vi "dllpathselect.vi"() -> (3 "appended path":path)   [LabVIEW 2025]
panel:
  out "number of replacements":i32
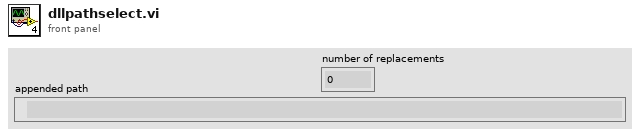
[diagram p1: front panel]
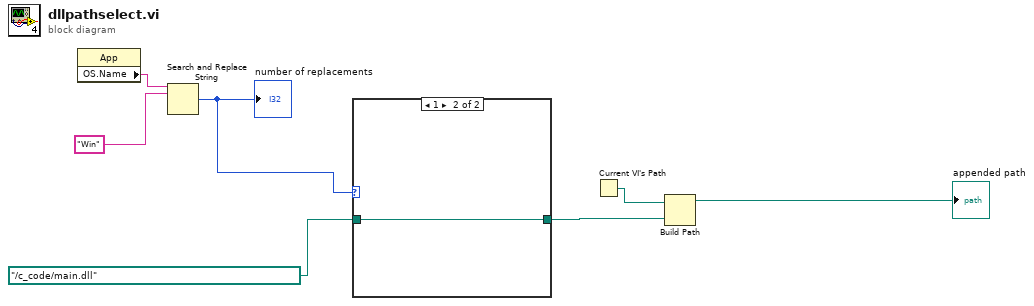
[diagram p0: block diagram]
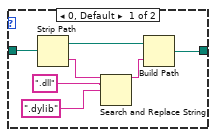
[diagram p2: hidden frame]
diagram:
  n1 = property class="App"() -> ("OS.Name"=w5:string)  [unwired: 2 in, 2 out]
  n2 = Search and Replace String(input string=w5, search string="Win") -> (number of replacements=w2:i32)  [unwired: 6 in, 3 out]
  "number of replacements" <- w2
  n3 = case shown="1" w2 {
    tunnel: path "../c_code/main.dll" ("name or relative path") -> [w14 w15]
    tunnel: [w8 w15] -> w3
    frame 0, Default {
      n4 = Strip Path(path=w14) -> (stripped path=w9:path, name=w13:string)
      n5 = Search and Replace String(input string=w13, search string=".dll", replace string=".dylib" ("replace string (\"\")")) -> (result string=w10:string)  [unwired: 5 in, 3 out]
      n6 = Build Path(base path=w9, name or relative path=w10) -> (appended path=w8:path)
    }
    frame 1 {
    }
  }
  n7 = Current VI's Path() -> (path=w7:path)
  n8 = Build Path(base path=w7, name or relative path=w3) -> (appended path=→"appended path":path)
